vi "hexatodecimal trials.vi"() -> ()   [LabVIEW 2019]
panel:
  out "*(type *) &x":string
  out "output string":string
  out "value":u8
  out "offset past number":i32
  in  "default (0 U32)":u8
  in  "string":string
  out "substring":string
  out "Data in Decimal":u8
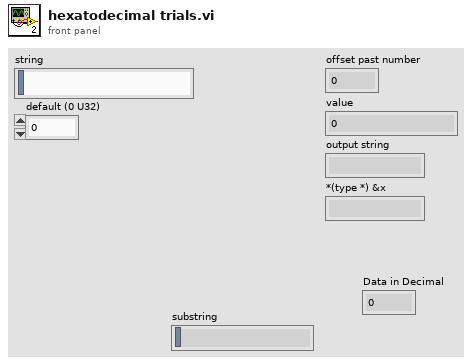
[diagram p1: front panel]
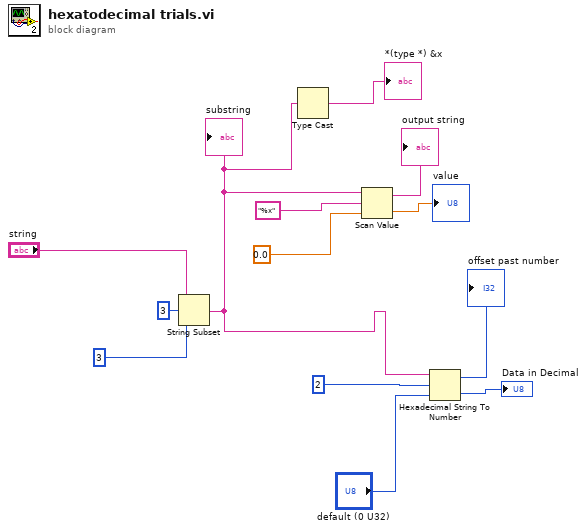
[diagram p0: block diagram]
diagram:
  n1 = String Subset(string="string", offset (0)=3, length (rest)=3 ("length (rest)")) -> (substring=w1:string)
  "substring" <- w1
  n2 = Type Cast(x=w1) -> (*(type *) &x=→"*(type *) &x":string)  [unwired: 1 in]
  n3 = Scan Value(string=w1, format string="%x", default (0 dbl)=0.0) -> (output string=→"output string":string, value=→"value":dbl)
  n4 = Hexadecimal String To Number(string=w1, offset=2, default (0uL)="default (0 U32)") -> (offset past number=→"offset past number":i32, number=→"Data in Decimal":u8)
